vi "Read Data.vi"(8 "error in (no error)":errorcluster, 11 "Data Cluster":T1={"Status"="", "Data sources"=[], "Data Names"=[], "Host name or address"="localhost", "Remote port"=35536, "Local port"=35535, "Key"="", "connection ID"=refnum}) -> (0 "error in (no error) 2":errorcluster, 1 "Array":dbl[](array[numeric]))   [LabVIEW 2014, in "get_data_mapper.lvlib"]
uses:
  get_data_mapper.lvlib
  Module Data--cluster.ctl
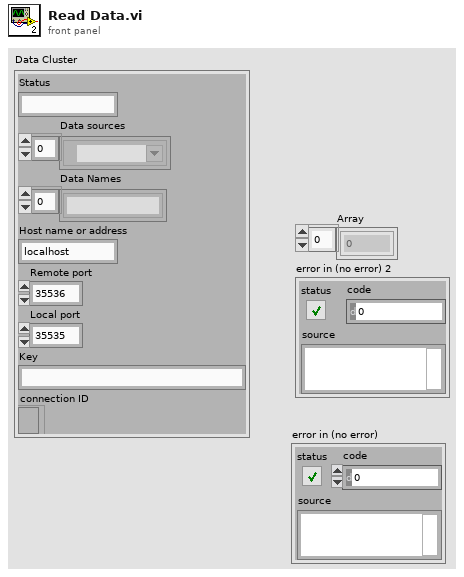
[diagram p1: front panel]
types:
  T1 = typedef "get_data_mapper.lvlib/Module Data--cluster.ctl" = cluster{"Status":string, "Data sources":refnum<k21>[], "Data Names":string[], "Host name or address":string, "Remote port":u16, "Local port":u16, "Key":string, "connection ID":refnum<k16>}
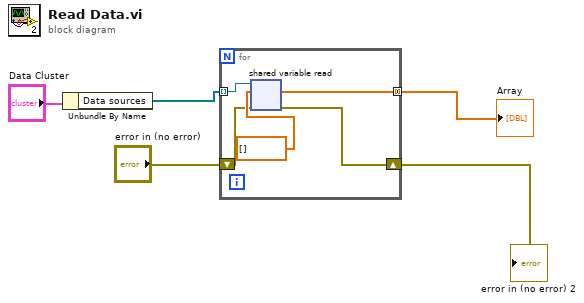
[diagram p0: block diagram]
diagram:
  n1 = Unbundle By Name("Data Cluster") -> ("Data sources"=w4:refnum<k21>[])
  n2 = for {
    tunnel: w4 -> [w10] mode=indexing
    tunnel: [w8] -> w3 mode=concatenating
    shift-right: [w6] -> w1
    shift-left: "error in (no error)" -> [w7]
    n3 = shared-variable-read(w10, w7, dbl[] []) -> (w6:errorcluster, w8:dbl[])  [unwired: 2 out]
  }
  "Array" <- w3
  "error in (no error) 2" <- w1
